vi "Spawn Actor.vi"(7 "Actor in":refnum<class "Actor.lvclass">, 10 "Spawn":refnum<class "Spawn.lvclass">) -> (0 "Error out":errorcluster, 5 "Actor out":refnum<class "Actor.lvclass">)   [LabVIEW 2025, in "jettl.lvlib" / "Actor.lvlib" / "Core Actor.lvclass"]
uses:
  Core Actor.lvclass
  Actor/Actor.lvclass
  Spawn/Spawn/Spawn.lvclass
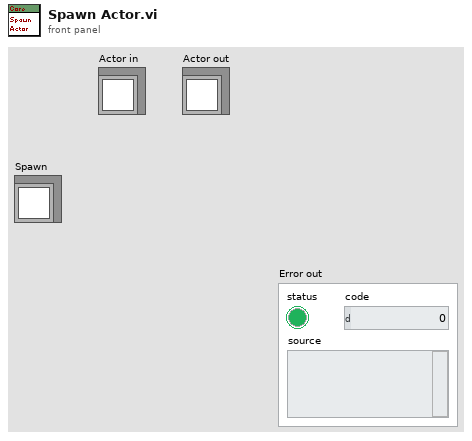
[diagram p1: front panel]
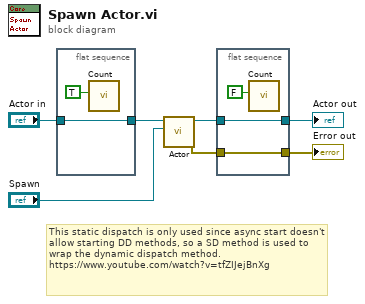
[diagram p0: block diagram]
diagram:
  # "This static dispatch is only used since async start doesn't allow starting DD methods, so a SD method is used to wrap the dynamic dispatch method.\nhttps://www.youtube.com/watch?v=tfZIJejBnXg"
  n1 = flat-sequence {
    tunnel: [w8] -> w4
    tunnel: "Actor in" -> [w8]
    frame #0 {
      n2 = call "Count.vi"("Increment?"=TRUE) -> ()  [unwired: 11 in]
    }
  }
  n3 = call-dynamic "Actor.vi"("Spawn"="Spawn", "Actor in"=w4) -> ("Error out"=w5:errorcluster, "Actor out"=w6:refnum<class "Actor.lvclass">)  [unwired: 8 in]
  n4 = flat-sequence {
    tunnel: [w11] -> w7
    tunnel: w5 -> [w11]
    tunnel: [w10] -> w3
    tunnel: w6 -> [w10]
    frame #0 {
      n5 = call "Count.vi"("Increment?"=FALSE) -> ()  [unwired: 11 in]
    }
  }
  "Error out" <- w7
  "Actor out" <- w3
